vi "Read Density.vi"(8 "error in (no error)":errorcluster, 11 "Bronkhorst Settings in":T1={"VISA resource name"="", "Simulated?"=FALSE, "Smoothing Steps"=1} {"Smoothing Steps" min=1 step=1}) -> (0 "error out":errorcluster, 1 "Connection Error":bool, 2 "Density kg/m^3":sgl, 3 "Bronkhorst Settings out":T1={"VISA resource name"="", "Simulated?"=FALSE, "Smoothing Steps"=1} {"Smoothing Steps" min=1 step=1})   [LabVIEW 2018, in "Bronkhorst M13 Flow Meter.lvlib"]
uses:
  Bronkhorst M13 Flow Meter.lvlib
  Settings Cluster.ctl
  <vilib>/regexp/Match Regular Expression.xnode
  <vilib>/ptbypt/NI_PtbyPt.lvlib
panel:
  out "whole match":string
  out "read buffer":string
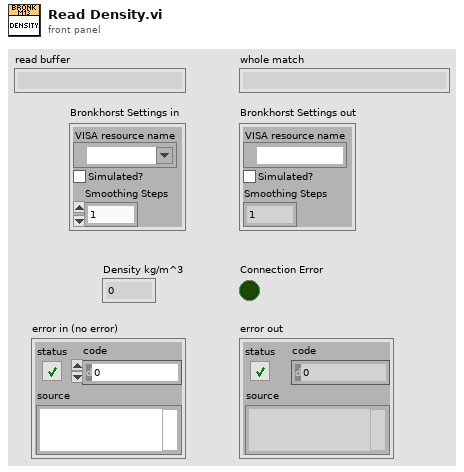
[diagram p1: front panel]
types:
  T1 = typedef "Bronkhorst M13 Flow Meter.lvlib/Settings Cluster.ctl" = cluster{"VISA resource name":refnum<visa-resource-name>, "Simulated?":bool, "Smoothing Steps":i32}
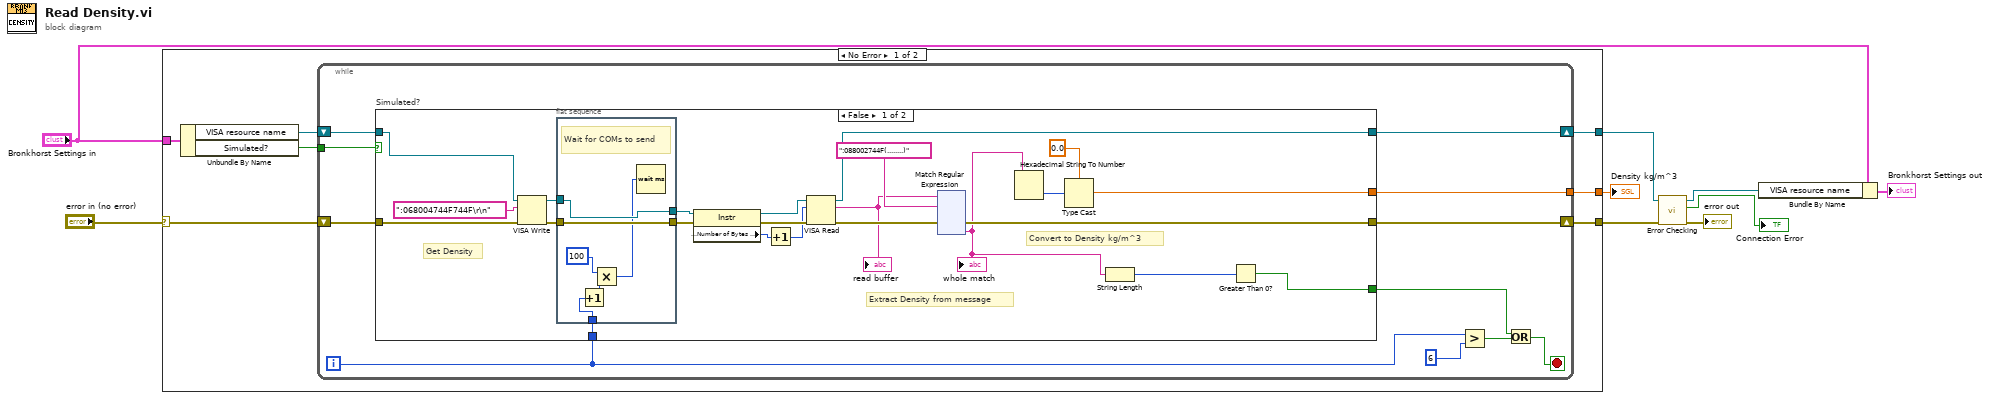
[diagram p0: block diagram]
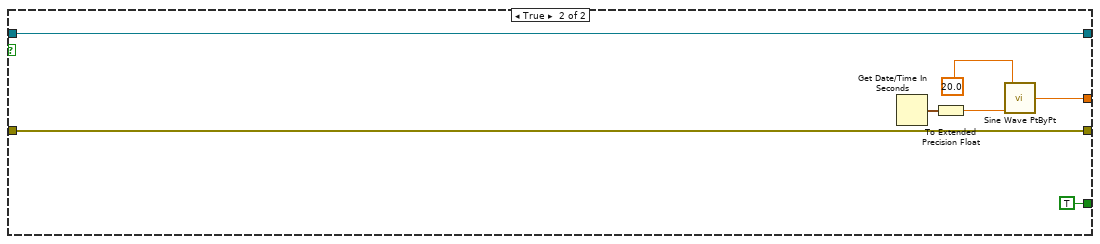
[diagram p2: hidden frame]
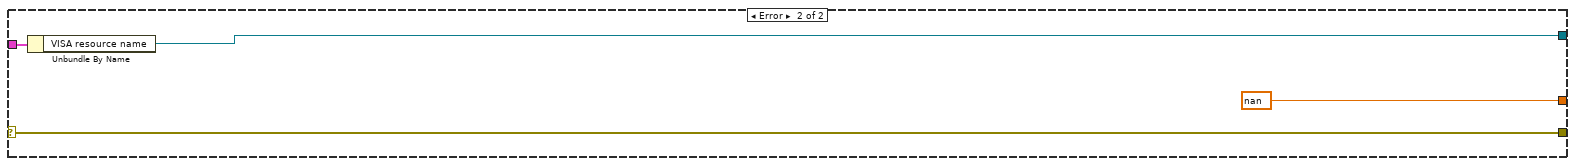
[diagram p3: hidden frame]
diagram:
  n1 = case shown="No Error" "error in (no error)" {
    selector: "error in (no error)" -> [w15 w183]
    tunnel: [w14 w183] -> w4
    tunnel: "Bronkhorst Settings in" -> [w13 w182]
    tunnel: [w11 w181] -> w6
    tunnel: [w10 nan ("sine wave")] -> w1
    frame No Error {
      n2 = Unbundle By Name(w13) -> ("VISA resource name"=w12:refnum<visa-resource-name>, "Simulated?"=w16:bool)
      n3 = while {
        tunnel: w16 -> [w27]
        tunnel: [w22] -> w10
        shift-right: [w25] -> w14
        shift-left: w15 -> [w26]
        shift-right: [w23] -> w11
        shift-left: w12 -> [w24]
        i -> [w17]
        stop <- w21 stop-if-true
        n4 = case "Simulated?" shown="False" w27 {
          tunnel: [w33 w179] -> w25
          tunnel: w26 -> [w42 w179]
          tunnel: [w39 w175] -> w23
          tunnel: w24 -> [w43 w175]
          tunnel: [w36 w174] -> w22
          tunnel: [w28 TRUE] -> w20
          tunnel: w17 -> [w31 _]
          frame False {
            # "Extract Density from message"
            # "Get Density"
            # "Convert to Density kg/m^3"
            n5 = VISA Write(VISA resource name=w43, write buffer=":068004744F744F\r\n" ("Command"), error in (no error)=w42) -> (VISA resource name out=w47:refnum<visa-resource-name>, error out=w45:errorcluster)  [unwired: 1 out]
            n6 = flat-sequence {
              tunnel: [w172] -> w46
              tunnel: w47 -> [w172]
              tunnel: [w171] -> w44
              tunnel: w45 -> [w171]
              tunnel: w31 -> [w168]
              frame #0 {
                # "Wait for COMs to send"
                n7 = Increment(x=w168) -> (x+1=w167:i32)
                n8 = Multiply(x=u32 100 ("milliseconds to wait"), y=w167) -> (x*y=w169:u32)
                n9 = Wait (ms)(milliseconds to wait=w169) -> ()  [unwired: 1 out]
              }
            }
            n10 = property class="Instr"(reference=w46, error in=w44) -> (reference out=w49:refnum<visa-resource-name>, error out=w48:errorcluster, "Serial Settings:Number of Bytes at Serial Port"=w41:u32)
            n11 = Increment(x=w41) -> (x+1=w40:u32)
            n12 = VISA Read(VISA resource name=w49, byte count=w40, error in (no error)=w48) -> (VISA resource name out=w39:refnum<visa-resource-name>, read buffer=w30:string, error out=w34:errorcluster)  [unwired: 1 out]
            "read buffer" <- w30
            n13 = xnode "Match Regular Expression"("input string"=w30, "regular expression"=":088002744F(........)" ("Regular Expression for Extracting Weight"), "error in"=w34) -> ("error out"=w33:errorcluster, "submatch 1"=w32:string)  [unwired: 3 in, 4 out]
            "whole match" <- w32
            n14 = Hexadecimal String To Number(string=w32) -> (number=w37:u32)  [unwired: 2 in, 1 out]
            n15 = Type Cast(type=sgl 0.0, x=w37) -> (*(type *) &x=w36:sgl)
            n16 = String Length(string=w32) -> (length=w29:i32)
            n17 = Greater Than 0?(x=w29) -> (x > 0?=w28:bool)
          }
          frame True {
            n18 = Get Date/Time In Seconds() -> (seconds since 1Jan1904=w178:timestamp)
            n19 = To Extended Precision Float(1:w178) -> (0:w177:ext)
            n20 = call <vilib>:"Sine Wave PtByPt.vi"("time"=w177, "amplitude"=20.0) -> ("sine wave"=w174:dbl)  [unwired: 2 in]
          }
        }
        n21 = Greater?(x=w17, y=6) -> (0:w18:bool)
        n22 = Or(x=w20, y=w18) -> (x .or. y?=w21:bool)
      }
    }
    frame Error {
      n23 = Unbundle By Name(w182) -> ("VISA resource name"=w181:refnum<visa-resource-name>)
    }
  }
  "Density kg/m^3" <- w1
  n24 = call "Error Checking.vi"("error in (no error)"=w4, "VISA resource name"=w6) -> ("error out"=→"error out":errorcluster, "Connection Error"=→"Connection Error":bool, "VISA resource name"=w5:refnum<visa-resource-name>)  [unwired: 7 in]
  n25 = Bundle By Name(cluster="Bronkhorst Settings in", "VISA resource name"=w5) -> (→"Bronkhorst Settings out":T1)
